vi "AIM664 Transmit 2.vi"() -> ()   [LabVIEW 2020]
uses:
  AIM664LV.lvlib
panel:
  out "error out":errorcluster
  in  "TxQueueWriteIn":T1={"HeaderType"=0, "EntryCount"=1, "WriteBytes"=150, "FrameSize"=64, "FrameType"=0, "InterFrameGap"=1000, "PacketGroupWaitTime"=0, "PayloadBufferMode"=0, "PayloadGenerationMode"=0, "BufferQueueHandle"=0, "ExternalStrobe"=0, "PreambleCount"=0, "Skew"=1, "NetSelect"=0, "FrameStartMode"=0, "PhysErrorInjection"=0, "SequenceNumberInit"=65535, "SequenceNumberOffset"=65535, "Code"=0, "Interrupt"=0, "Data"=[3, 0, 0, 0, 0, 0, 2, 0, 0, 1, 1, 32, 8, 0, 69, 0, 0, 45, 0, 0, 64, 0, 1, 17, 141, 223, 10, 1, 1, 0, 224, 224, 0, 0, 0, 1, 0, 2, 0, 25, 0, 0, 65, 66, 67, 68, 69, 70, 71, 72, 73, 74, 75, 76, 77, 78, 79, 80, 81, 11]} {"Data" format="%x"; "FrameType" items=["FDX_TX_FRAME_STD", "FDX_TX_FRAME_INSTR"]; "SequenceNumberOffset" items=["FDX_TX_FRAME_SEQ_OFFS_AUTO "=65535]; "SequenceNumberInit" items=["FDX_TX_FRAME_SEQ_INIT_AUTO"=65535]; "PhysErrorInjection" items=["FDX_TX_FRAME_ERR_OFF"=0, "FDX_TX_FRAME_ERR_CRC"=1, "FDX_TX_FRAME_ERR_ALI"=2, "FDX_TX_FRAME_ERR_PRE"=4, "FDX_TX_FRAME_ERR_PHY"=8]; "FrameStartMode" items=["FDX_TX_FRAME_START_IFG", "FDX_TX_FRAME_START_PGWT", "FDX_TX_FRAME_START_TRG"]; "NetSelect" items=["FDX_TX_FRAME_DLY_A"=0, "FDX_TX_FRAME_DLY_B"=1, "FDX_TX_FRAME_BOTH "=3, "FDX_TX_FRAME_ONLY_A"=4, "FDX_TX_FRAME_ONLY_B "=5]; "PreambleCount" max=15; "ExternalStrobe" items=["FDX_DIS", "FDX_ENA"]; "PayloadGenerationMode" items=["FDX_TX_FRAME_PGM_USER"=0, "FDX_TX_FRAME_PGM_IP_PART"=1, "FDX_TX_FRAME_PGM_IP_FULL"=2, "FDX_TX_FRAME_PGM_IP_PART_TT"=10, "FDX_TX_FRAME_PGM_IP_FULL_TT"=20]; "PayloadBufferMode" items=["FDX_TX_FRAME_PBM_STD", "FDX_TX_FRAME_PBM_MAC", "FDX_TX_FRAME_PBM_UDP"]; "HeaderType" items=["FDX_TX_FRAME_HEADER_GENERIC ", "FDX_TX_FRAME_HEADER_REPLAY"]}
  out "Board Control Out":T2={"PortConfig"=[0, 0, 4294967295, 4294967295], "PortSpeed"=[0, 0, 4294967295, 4294967295], "PortUsed"=[4, 0, 0, 0], "PortGoodLink"=[1, 1, 4294967295, 4294967295], "ExpertMode"=[0, 0, 4294967295, 4294967295], "GlobalMemFree"=41940624, "SharedMemFree"=16564184, "RxVeriMode"=0} {"SharedMemFree" format="%x"; "GlobalMemFree" format="%x"; "ExpertMode" items=["FDX_EXPERT_MODE", "FDX_DISA_GHOST"]; "PortGoodLink" items=["FDX_NO_LINK", "FDX_GOOD_LINK"]; "PortSpeed" items=["FDX_100MBIT", "FDX_10MBIT", "FDX_AUTO_100MBIT", "FDX_AUTO_10MBIT"]; "PortConfig" items=["FDX_SINGLE", "FDX_REDUNDANT"]}
  in  "BoardControlIn":T3={"Control"=1, "Port1ConfigIn"=0, "Port2ConfigIn"=0, "Port3ConfigIn"=0, "Port4ConfigIn"=0, "Port1SpeedIn"=0, "Port2SpeedIn"=0, "Port3SpeedIn"=0, "Port4SpeedIn"=0, "Expert1Mode"=0, "Expert2Mode"=0, "Expert3Mode"=0, "Expert4Mode"=0, "RxVeriModeIn"=0, "RxVeriData1"=0, "RxVeriData2"=0, "RxVeriData3"=0, "RxVeriData4"=0, "RxVeriData5"=0, "RxVeriData6"=0, "RxVeriData7"=0, "RxVeriData8"=0, "RxVeriMask1"=0, "RxVeriMask2"=0, "RxVeriMask3"=0, "RxVeriMask4"=0, "RxVeriMask5"=0, "RxVeriMask6"=0, "RxVeriMask7"=0, "RxVeriMask8"=0} {"Expert4Mode" items=["FDX_EXPERT_MODE", "FDX_DISA_GHOST"]; "Expert3Mode" items=["FDX_EXPERT_MODE", "FDX_DISA_GHOST"]; "Expert2Mode" items=["FDX_EXPERT_MODE", "FDX_DISA_GHOST"]; "Expert1Mode" items=["FDX_EXPERT_MODE", "FDX_DISA_GHOST"]; "Port4SpeedIn" items=["FDX_100MBIT", "FDX_10MBIT", "FDX_AUTO_100MBIT", "FDX_AUTO_10MBIT"]; "Port3SpeedIn" items=["FDX_100MBIT", "FDX_10MBIT", "FDX_AUTO_100MBIT", "FDX_AUTO_10MBIT"]; "Port2SpeedIn" items=["FDX_100MBIT", "FDX_10MBIT", "FDX_AUTO_100MBIT", "FDX_AUTO_10MBIT"]; "Port1SpeedIn" items=["FDX_100MBIT", "FDX_10MBIT", "FDX_AUTO_100MBIT", "FDX_AUTO_10MBIT"]; "Port4ConfigIn" items=["FDX_SINGLE", "FDX_REDUNDANT"]; "Port3ConfigIn" items=["FDX_SINGLE", "FDX_REDUNDANT"]; "Port2ConfigIn" items=["FDX_SINGLE", "FDX_REDUNDANT"]; "Port1ConfigIn" items=["FDX_SINGLE", "FDX_REDUNDANT"]; "Control" items=["FDX_READ", "FDX_WRITE"]}
  out "ResourceInfo 2":T4 {"PortMode" items=[" FDX_SINGLE", "FDX_REDUNDANT"]}
  out "ResourceInfo":T4 {"PortMode" items=[" FDX_SINGLE", "FDX_REDUNDANT"]}
  in  "Input Cluster 2":T5 {"ExtendedStopMode" items=["FDX_ESTOP_NOT_USED", "FDX_ESTOP_EXT_TRG", "FDX_ESTOP_EXT_TRG_RESTART", "FDX_ESTOP_TIME"]; "StartMode" items=["FDX_STOP", "FDX_START", "FDX_START_TRG", "FDX_START_TIME"]}
  in  "Input Cluster":T5={"StartMode"=1, "Count"=100, "Sign"=0, "Day"=0, "Hour"=0, "Min"=0, "Second"=0, "MilliSec"=0, "MicroSec"=0, "ExtendedStopMode"=0, "TransmitTime"=0} {"ExtendedStopMode" items=["FDX_ESTOP_NOT_USED", "FDX_ESTOP_EXT_TRG", "FDX_ESTOP_EXT_TRG_RESTART", "FDX_ESTOP_TIME"]; "StartMode" items=["FDX_STOP", "FDX_START", "FDX_START_TRG", "FDX_START_TIME"]}
  out "Output Cluste":cluster{"QueueBaseAddr":u32, "QueueSizeOut":u32}={"QueueBaseAddr"=25168256, "QueueSizeOut"=4194304}
  in  "QueueSizeIn":u32
  in  "Input Cluster":T6={"SrvName"="local", "ClHostName"="local", "ClUser"="Brett", "ClApplication"="Test", "ClApplicationVersion"="V01.00", "ResourceID"=1, "Privileges"=4294967295} {"Privileges" items=["PRIVILEGES_ADMIN"=4294967295]}
  in  "Input Cluster":T7={"SrvName"="local", "ResourceID"=1, "ResourceType"=0} {"ResourceType" items=["Board", "Port"]}
  out "Output Cluster 2":T8={"ResourceID"=1, "ResourceType"=0, "ResourceInfo"="AMC-FDX-2", "StructId"=0}
  in  "ServerRElement":u32=1
  in  "PortMap":u32
  out "Output Cluster":T9={"PortConfig"=0, "PortUsed"=4, "GlobalMemFree"=46135008, "SharedMemFree"=16564184} {"PortConfig" items=["FDX_SINGLE", "FDX_REDUNDANT"]}
  out "Output Cluster":T10={"TxStatus"=100, "Frames"=1, "TransmitMode"=0, "FramesPortB"=0} {"TransmitMode" items=["FDX_TX_GENERIC", "FDX_TX_REPLAY", "FDX_TX_INDIVIDUAL"]; "TxStatus" items=["FDX_STAT_STOP", "FDX_STAT_RUN", "FDX_STAT_ERROR", "FDX_STAT_WAIT_F_TRIG"]}
  in  "RerosPortDelay":u32
  in  "TransmitMode":u32(ring) items=["FDX_TX_GENERIC", "FDX_TX_REPLAY", "FDX_TX_INDIVIDUAL"]
  in  "Input Cluster":T7={"SrvName"="local", "ResourceID"=2, "ResourceType"=1} {"ResourceType" items=["Board", "Port"]}
  in  "Input Cluster":T6={"SrvName"="local", "ClHostName"="local", "ClUser"="Brett", "ClApplication"="Test", "ClApplicationVersion"="V01.00", "ResourceID"=2, "Privileges"=4294967295} {"Privileges" items=["PRIVILEGES_ADMIN"=4294967295]}
  out "Output Cluster":T8={"ResourceID"=2, "ResourceType"=1, "ResourceInfo"="Port1", "StructId"=0}
  in  "ServerRElement":u32=2
  out "NuOfResources":u32=3
  in  "SrvName":string="local"
  out "NuOfServers":u32=1
  # "ARINC 664 Transmit Data"
  # "Overview: Configure the board to Transmit Data.\nRequirement: At least one AIM ARINC-664 board with installed AIM ARINC 664 BSP.\nRestrictions: None.\nInstruction:\n1. Run the VI.\n2. Verify the results in the controls and indicators."
  # "Tx Port"
  # "Board"
  # "Tx Port"
  # "Board"
  # "FdxMonGetStatusCvii"
  # "FdxRxControlCvi"
  # "FdxInitCvi"
  # "FdxLogoutCvi"
  # "CountServerResourcesCvi"
  # "GetServerResourcesCvi"
  # "QueryServerResourceCvi"
  # "FdxLoginCvi"
  # "FdxBoardControlCvi"
  # "FdxTxModeControlCvi"
  # "FdxTxQueueCreateCvi"
  # "FdxLogoutCvi"
  # "GetServerResourcesCvi"
  # "QueryServerResourceCvi"
  # "FdxTxPortInitCvi"
  # "FdxTxQueueWriteCvi"
  # "FdxTxControlCvi"
  # "FdxTxStatusCvi"
  # "FdxTxControlCvi"
  # "FdxLoginCvi"
  # "Input"
  # "Input"
  # "Input"
  # "Input"
  # "Input"
  # "Input"
  # "Input"
  # "Input"
  # "Input"
  # "Input"
  # "Input"
  # "Input"
  # "Input"
  # "Output"
  # "Input"
  # "Input"
  # "Input"
  # "Input"
  # "Input"
  # "Output"
  # "Output"
  # "Output"
  # "Output"
  # "Output"
  # "Output"
  # "Output"
  # "Output"
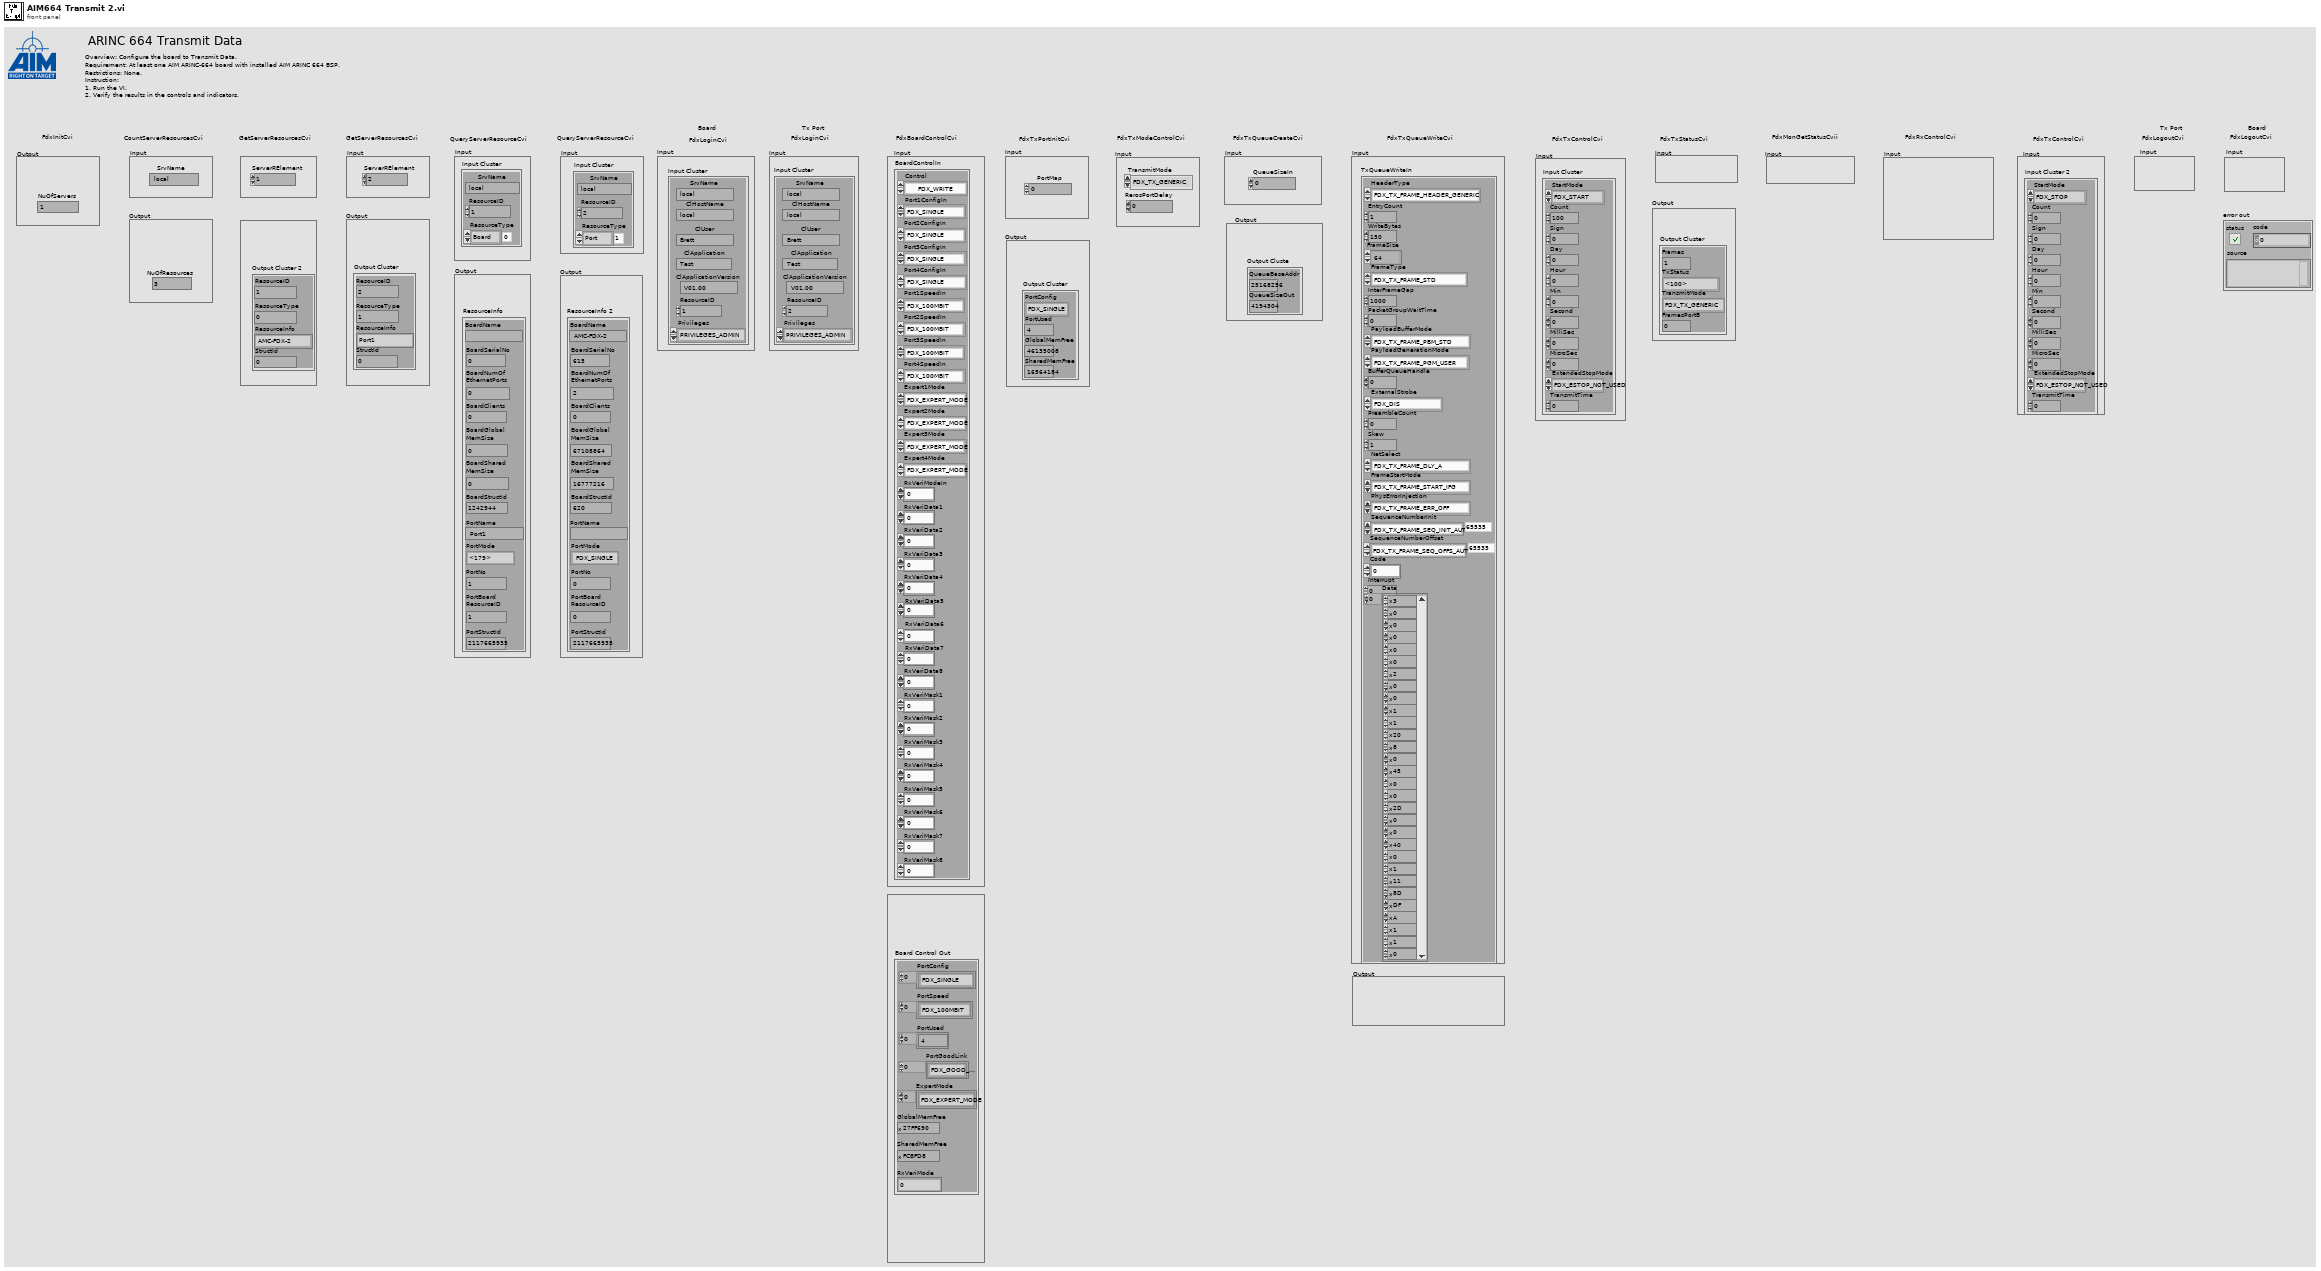
[diagram p1: front panel]
types:
  T1 = cluster{"HeaderType":u32, "EntryCount":u32, "WriteBytes":u32, "FrameSize":u16, "FrameType":u8, "InterFrameGap":u32, "PacketGroupWaitTime":u32, "PayloadBufferMode":u8, "PayloadGenerationMode":u8, "BufferQueueHandle":u32, "ExternalStrobe":u8, "PreambleCount":u8, "Skew":u32, "NetSelect":u8, "FrameStartMode":u8, "PhysErrorInjection":u32, "SequenceNumberInit":u16, "SequenceNumberOffset":u16, "Code":u8, "Interrupt":u8, "Data":u8[]}
  T2 = cluster{"PortConfig":u32[], "PortSpeed":u32[], "PortUsed":u32[], "PortGoodLink":u32[], "ExpertMode":u32[], "GlobalMemFree":u32, "SharedMemFree":u32, "RxVeriMode":u32}
  T3 = cluster{"Control":u32, "Port1ConfigIn":u32, "Port2ConfigIn":u32, "Port3ConfigIn":u32, "Port4ConfigIn":u32, "Port1SpeedIn":u32, "Port2SpeedIn":u32, "Port3SpeedIn":u32, "Port4SpeedIn":u32, "Expert1Mode":u32, "Expert2Mode":u32, "Expert3Mode":u32, "Expert4Mode":u32, "RxVeriModeIn":u32, "RxVeriData1":u32, "RxVeriData2":u32, "RxVeriData3":u32, "RxVeriData4":u32, "RxVeriData5":u32, "RxVeriData6":u32, "RxVeriData7":u32, "RxVeriData8":u32, "RxVeriMask1":u32, "RxVeriMask2":u32, "RxVeriMask3":u32, "RxVeriMask4":u32, "RxVeriMask5":u32, "RxVeriMask6":u32, "RxVeriMask7":u32, "RxVeriMask8":u32}
  T4 = cluster{"BoardName":string, "BoardSerialNo":u32, "BoardNumOf\nEthernetPorts":u32, "BoardClients":u32, "BoardGlobal\nMemSize":u32, "BoardShared\nMemSize":u32, "BoardStructId":u32, "PortName":string, "PortMode":u32, "PortNo":u32, "PortBoard\nResourceID":u32, "PortStructId":u32}
  T5 = cluster{"StartMode":i32, "Count":u32, "Sign":i32, "Day":u32, "Hour":u32, "Min":u32, "Second":u32, "MilliSec":u32, "MicroSec":u32, "ExtendedStopMode":i32, "TransmitTime":u32}
  T6 = cluster{"SrvName":string, "ClHostName":string, "ClUser":string, "ClApplication":string, "ClApplicationVersion":string, "ResourceID":u32, "Privileges":u32}
  T7 = cluster{"SrvName":string, "ResourceID":u32, "ResourceType":u32}
  T8 = cluster{"ResourceID":u32, "ResourceType":u32, "ResourceInfo":string, "StructId":u32}
  T9 = cluster{"PortConfig":u32, "PortUsed":u32, "GlobalMemFree":u32, "SharedMemFree":u32}
  T10 = cluster{"TxStatus":i32, "Frames":u32, "TransmitMode":u32, "FramesPortB":u32}
  T11 = typedef "AIM664LV.lvlib/port_configuration.ctl" = u32
  T12 = typedef "AIM664LV.lvlib/port_speed.ctl" = u32
  T13 = typedef "AIM664LV.lvlib/port_condition.ctl" = u32
  T14 = typedef "AIM664LV.lvlib/expert_mode.ctl" = u32
  T15 = cluster{"PortConfig":T11[], "PortSpeed":T12[], "PortUsed":u32[], "PortGoodLink":T13[], "ExpertMode":T14[], "GlobalMemFree":u32, "SharedMemFree":u32, "RxVeriMode":u32}
  T16 = cluster{"TxStatus":u32, "Frames":u32, "TransmitMode":u32, "FramesPortB":u32}
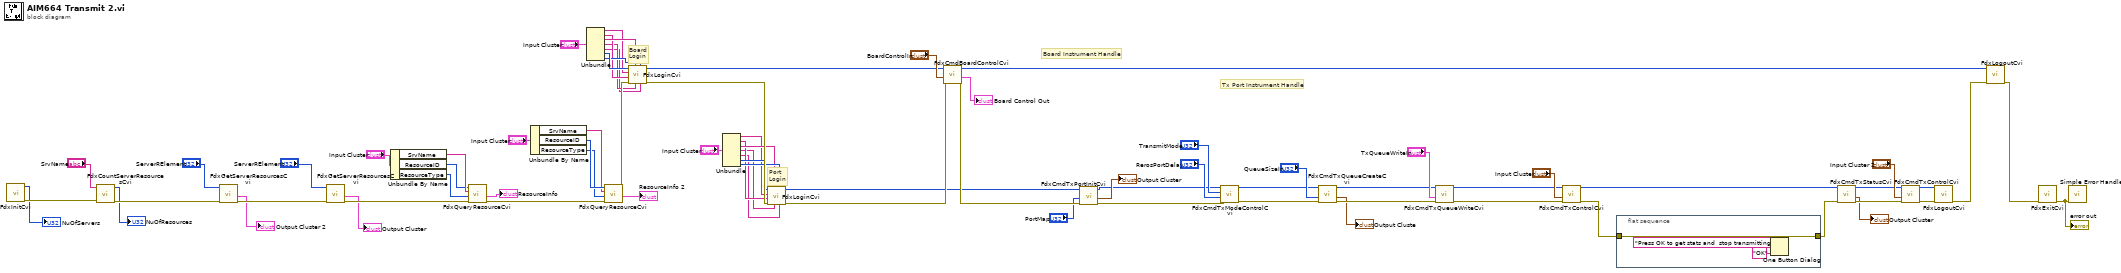
[diagram p0: block diagram]
diagram:
  # "Tx Port Instrument Handle"
  # "Board Instrument Handle"
  # "Port\nLogin"
  # "Board\nLogin"
  n1 = call "FdxInitCvi.vi"() -> ("error out"=w71:errorcluster, "Number of Servers"=→"NuOfServers":u32)  [unwired: 10 in]
  n2 = call "FdxCountServerResourcesCvi.vi"("error in"=w71, "SrvName (local)"="SrvName") -> ("error out"=w70:errorcluster, "Number of Resources"=→"NuOfResources":u32)  [unwired: 8 in]
  n3 = call "FdxGetServerResourcesCvi.vi"("error in"=w70, "ServerRElement"="ServerRElement") -> ("error out"=w69:errorcluster, "ServerResourceInfo"=→"Output Cluster 2":T8)  [unwired: 4 in, 4 out]
  n4 = call "FdxGetServerResourcesCvi.vi"("error in"=w69, "ServerRElement"="ServerRElement") -> ("error out"=w75:errorcluster, "ServerResourceInfo"=→"Output Cluster":T8)  [unwired: 4 in, 4 out]
  n5 = Unbundle By Name("Input Cluster") -> ("SrvName"=w34:string, "ResourceID"=w33:u32, "ResourceType"=w32:u32)
  n6 = call "FdxQueryResourceCvi.vi"("error in"=w75, "ResourceType"=w32, "SrvName"=w34, "ResourceID"=w33) -> ("error out"=w68:errorcluster, "ResourceInfo"=→"ResourceInfo":T4)  [unwired: 5 in, 1 out]
  n7 = Unbundle By Name("Input Cluster") -> ("SrvName"=w29:string, "ResourceID"=w30:u32, "ResourceType"=w28:u32)
  n8 = Unbundle("Input Cluster") -> ("SrvName"=w23:string, "ClHostName"=w22:string, "ClUser"=w24:string, "ClApplication"=w21:string, "ClApplicationVersion"=w20:string, "ResourceID"=w26:u32, "Privileges"=w25:u32)
  n9 = call "FdxQueryResourceCvi.vi"("error in"=w68, "ResourceType"=w28, "SrvName"=w29, "ResourceID"=w30) -> ("error out"=w67:errorcluster, "ResourceInfo"=→"ResourceInfo 2":T4)  [unwired: 5 in, 1 out]
  n10 = call "FdxLoginCvi.vi"("ClApplicationVersion"=w20, "Privileges"=w25, "ClApplication"=w21, "ClUser"=w24, "error in"=w67, "ClHostName"=w22, "SrvName"=w23, "ResourceID"=w26) -> ("error out"=w66:errorcluster, "InstrumentHandle"=w11:u32)  [unwired: 2 in]
  n11 = Unbundle("Input Cluster") -> ("SrvName"=w15:string, "ClHostName"=w14:string, "ClUser"=w16:string, "ClApplication"=w13:string, "ClApplicationVersion"=w12:string, "ResourceID"=w18:u32, "Privileges"=w17:u32)
  n12 = call "FdxLoginCvi.vi"("ClApplicationVersion"=w12, "Privileges"=w17, "ClApplication"=w13, "ClUser"=w16, "error in"=w66, "ClHostName"=w14, "SrvName"=w15, "ResourceID"=w18) -> ("error out"=w59:errorcluster, "InstrumentHandle"=w9:u32)  [unwired: 2 in]
  n13 = call "FdxCmdBoardControlCvi.vi"("error in"=w59, "BoardControlIn (read)"="BoardControlIn", "InstrumentHandle_board in"=w11) -> ("error out"=w65:errorcluster, "Board Control Out"=→"Board Control Out":T15, "InstrumentHandle_board out"=w10:u32)  [unwired: 6 in]
  n14 = call "FdxCmdTxPortInitCvi.vi"("error in"=w65, "PortMap"="PortMap", "InstrumentHandle_port"=w9) -> ("error out"=w74:errorcluster, "PortInitOut"=→"Output Cluster":T9, "InstrumentHandle_port"=w8:u32)  [unwired: 6 in]
  n15 = call "FdxCmdTxModeControlCvi.vi"("error in"=w74, "RerosPortDelay"="RerosPortDelay", "TransmitMode"="TransmitMode", "InstrumentHandle_port"=w8) -> ("error out"=w64:errorcluster, "InstrumentHandle_port"=w7:u32)  [unwired: 6 in]
  n16 = call "FdxCmdTxQueueCreateCvi.vi"("error in"=w64, "QueueSizeIn"="QueueSizeIn", "InstrumentHandle_port"=w7) -> ("error out"=w63:errorcluster, "TxQueueInfo"=→"Output Cluste":cluster{"QueueBaseAddr":u32, "QueueSizeOut":u32}, "InstrumentHandle_port"=w6:u32)  [unwired: 6 in]
  n17 = call "FdxCmdTxQueueWriteCvi.vi"("error in"=w63, "TxQueueWriteIn"="TxQueueWriteIn", "InstrumentHandle_port"=w6) -> ("error out"=w58:errorcluster, "InstrumentHandle_port"=w5:u32)  [unwired: 7 in]
  n18 = call "FdxCmdTxControlCvi.vi"("error in"=w58, "TxControl"="Input Cluster", "InstrumentHandle_port"=w5) -> ("error out"=w73:errorcluster, "InstrumentHandle_port"=w4:u32)  [unwired: 7 in]
  n19 = flat-sequence {
    tunnel: w73 -> [w78]
    tunnel: [w78] -> w72
    frame #0 {
      n20 = One Button Dialog(message="Press OK to get stats and  stop transmitting", button name ("OK")="OK") -> ()  [unwired: 1 out]
    }
  }
  n21 = call "FdxCmdTxStatusCvi.vi"("error in"=w72, "InstrumentHandle_port"=w4) -> ("error out"=w62:errorcluster, "TxStatus"=→"Output Cluster":T16, "InstrumentHandle_port"=w3:u32)  [unwired: 7 in]
  n22 = call "FdxCmdTxControlCvi.vi"("error in"=w62, "TxControl"="Input Cluster 2", "InstrumentHandle_port"=w3) -> ("error out"=w60:errorcluster, "InstrumentHandle_port"=w2:u32)  [unwired: 7 in]
  n23 = call "FdxLogoutCvi.vi"("error in"=w60, "InstrumentHandle"=w2) -> ("error out"=w61:errorcluster)  [unwired: 9 in]
  n24 = call "FdxLogoutCvi.vi"("error in"=w61, "InstrumentHandle"=w10) -> ("error out"=w57:errorcluster)  [unwired: 9 in]
  n25 = call "FdxExitCvi.vi"("error in"=w57) -> ("error out"=w1:errorcluster)  [unwired: 10 in]
  "error out" <- w1
  n26 = call <vilib>:"Simple Error Handler.vi"("error in (no error)"=w1) -> ()  [unwired: 4 in, 5 out]
